vi "Write Current Limit.vi"(8 "error in":errorcluster, 10 "Current Limit (mA)":i32, 11 "VISA in":refnum<visa-resource-name>) -> (0 "error out":errorcluster, 2 "Output":string, 3 "VISA out":refnum<visa-resource-name>)   [LabVIEW 2018]
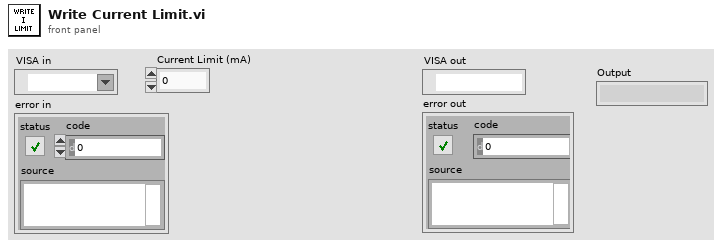
[diagram p1: front panel]
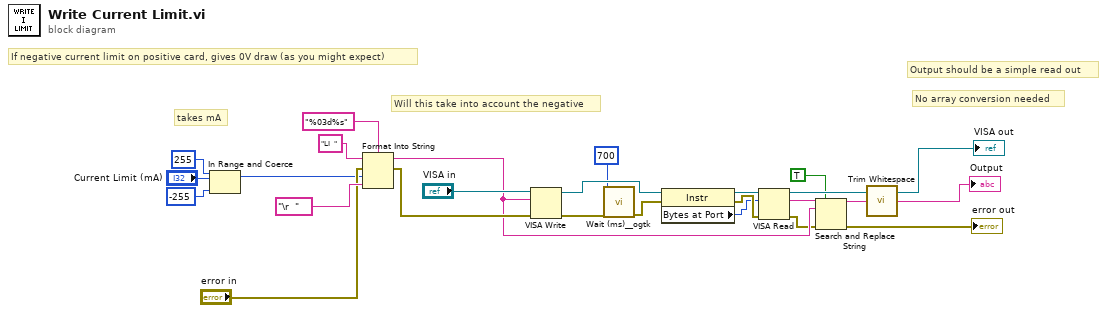
[diagram p0: block diagram]
diagram:
  # "Will this take into account the negative"
  # "takes mA"
  # "If negative current limit on positive card, gives 0V draw (as you might expect)"
  # "No array conversion needed"
  # "Output should be a simple read out"
  n1 = In Range and Coerce(upper limit=255, x="Current Limit (mA)", lower limit=-255) -> (coerced(x)=w1:i32)  [unwired: 1 out]
  n2 = Format Into String(format string="%03d%s", initial string="LI  ", error in="error in", w1, "\r  ") -> (resulting string=w7:string, error out=w9:errorcluster)
  n3 = VISA Write(VISA resource name="VISA in", write buffer=w7, error in (no error)=w9) -> (VISA resource name out=w21:refnum<visa-resource-name>, error out=w24:errorcluster)  [unwired: 1 out]
  n4 = call <userlib>:"Wait (ms)__ogtk.vi"("error in (no error)"=w24, "milliseconds to wait"=u32 700) -> ("error out"=w23:errorcluster)  [unwired: 8 in, 1 out]
  n5 = property class="Instr"(reference=w21, error in=w23) -> (reference out=w19:refnum<visa-resource-name>, error out=w22:errorcluster, "Bytes at Port"=w18:u32)
  n6 = VISA Read(VISA resource name=w19, byte count=w18, error in (no error)=w22) -> (VISA resource name out=→"VISA out":refnum<visa-resource-name>, read buffer=w8:string, error out=w4:errorcluster)  [unwired: 1 out]
  n7 = Search and Replace String(replace all?=TRUE ("replace all? (F)"), input string=w8, search string=w7, error in=w4) -> (result string=w6:string, error out=→"error out":errorcluster)  [unwired: 4 in, 2 out]
  n8 = call <vilib>:"Trim Whitespace.vi"("string"=w6) -> ("trimmed string"=→"Output":string)  [unwired: 1 in]
